vi "In range custom.vi"(9 "Lower limit":dbl, 10 "x":dbl, 11 "Upper limit":dbl) -> (3 "In range?":bool)   [LabVIEW 2018]
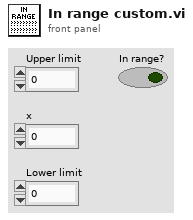
[diagram p1: front panel]
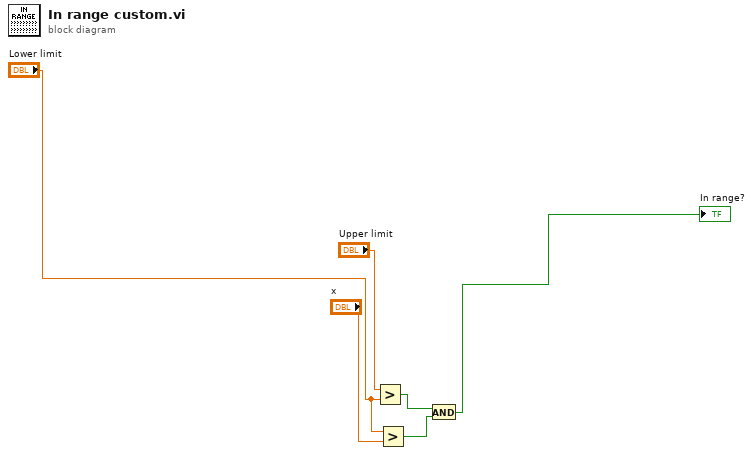
[diagram p0: block diagram]
diagram:
  n1 = Greater?(x="Upper limit", y="Lower limit") -> (0:w1:bool)
  n2 = Greater?(x="Lower limit", y="x") -> (0:w2:bool)
  n3 = And(x=w1, y=w2) -> (x .and. y?=→"In range?":bool)
